vi "Temperature Controller v1_0.vi"(0 "Set Point":dbl=50.0 format="%.3g", 1 "Present Value":dbl format="%.1g", 2 "Heater On/Off?":bool, 3 "Heater Pump":bool, 4 "Shut off":bool) -> (5 "Heater On":bool)   [LabVIEW 2012]
panel:
  in  "Tuning Parameters":T1={"Controller Gain, Kc"=45.0, "Reset Time, Ti (s)"=50.0, "Derivative Time, Td (s)"=10.0} {"Derivative Time, Td (s)" format="%.3g"; "Reset Time, Ti (s)" format="%.3g"; "Controller Gain, Kc" format="%.3g"}
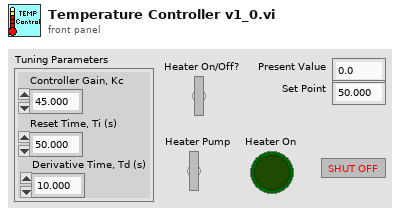
[diagram p1: front panel]
types:
  T1 = cluster{"Controller Gain, Kc":dbl, "Reset Time, Ti (s)":dbl, "Derivative Time, Td (s)":dbl}
  T2 = enum8{"Enabled", "Disabled", "Disabled and Grayed Out"}
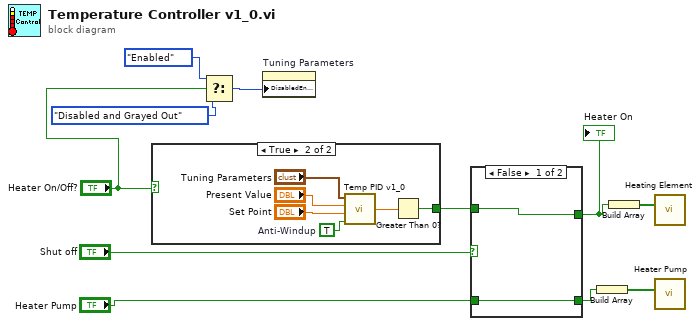
[diagram p0: block diagram]
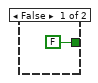
[diagram p2: hidden frame]
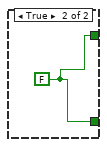
[diagram p3: hidden frame]
diagram:
  n1 = case shown="True" "Heater On/Off?" {
    tunnel: [FALSE w17] -> w4
    frame False {
    }
    frame True {
      w14 = TRUE  # Anti-Windup
      n2 = call "Temp PID v1_0.vi"("Anti-Windup"=w14, "Set Point"="Set Point", "Present Value"="Present Value", "Tuning Parameters"="Tuning Parameters") -> ("Controller Output"=w15:dbl)
      n3 = Greater Than 0?(x=w15) -> (x > 0?=w17:bool)
    }
  }
  n4 = Select(t=T2."Enabled" ("Disabled"), s="Heater On/Off?", f=T2."Disabled and Grayed Out" ("Disabled")) -> (s? t:f=w9:T2)
  n5 = property on="Tuning Parameters" class="Clust (strict)"("DisabledEnum"=w9) -> ()  [unwired: 2 in, 2 out]
  n6 = case shown="False" "Shut off" {
    tunnel: w4 -> [w19 _]
    tunnel: "Heater Pump" -> [w20 _]
    tunnel: [w20 w21] -> w2
    tunnel: [w19 w21] -> w1
    frame False {
    }
    frame True {
      w21 = FALSE
    }
  }
  "Heater On" <- w1
  n7 = Build Array(w2) -> (w6:bool[])
  n8 = Build Array(w1) -> (w5:bool[])
  n9 = call "Heating Element"("data"=w5) -> ()  [unwired: 17 in, 2 out]
  n10 = call "Heater Pump"("data"=w6) -> ()  [unwired: 17 in, 2 out]
